vi "TEMPLATE.vi"   [LabVIEW 2025, in "_Template.lvlib" / "Templates.lvlib" / "TEMPLATE jettl Actor.lvlib"]
uses:
  TEMPLATE jettl Actor.lvlib
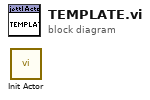
[diagram p0: block diagram]
diagram:
  n1 = call "Init Actor.vi"() -> ()  [unwired: 11 in, 1 out]
